vi "首页显示设置.vi"() -> ()   [LabVIEW 2016]
uses:
  <vilib>/Utility/config.llb/NI_LVConfig.lvlib
panel:
  in  "首页显示信息设置":T1={"水温"=FALSE, "pH"=FALSE, "DO"=FALSE, "Cond"=FALSE, "Turb"=FALSE, "氨氮"=FALSE, "总磷"=FALSE, "总氮"=FALSE, "CODMn"=FALSE, "CODCr"=FALSE, "水位"=FALSE, "流速"=FALSE, "瞬时流量"=FALSE, "室温"=TRUE, "湿度"=TRUE, "叶绿素a"=FALSE, "藻密度"=FALSE}
  in  "关闭":bool
  # "首页显示信息设置"
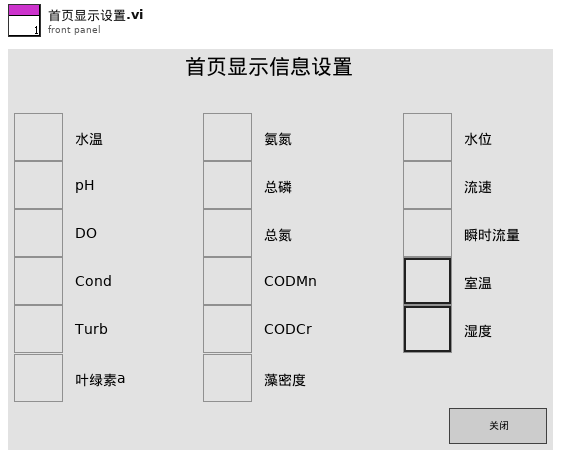
[diagram p1: front panel]
types:
  T1 = cluster{"水温":bool, "pH":bool, "DO":bool, "Cond":bool, "Turb":bool, "氨氮":bool, "总磷":bool, "总氮":bool, "CODMn":bool, "CODCr":bool, "水位":bool, "流速":bool, "瞬时流量":bool, "室温":bool, "湿度":bool, "叶绿素a":bool, "藻密度":bool}
  T2 = typedef "NI_LVConfig.lvlib/Config Data RefNum.ctl" = refnum<k1>
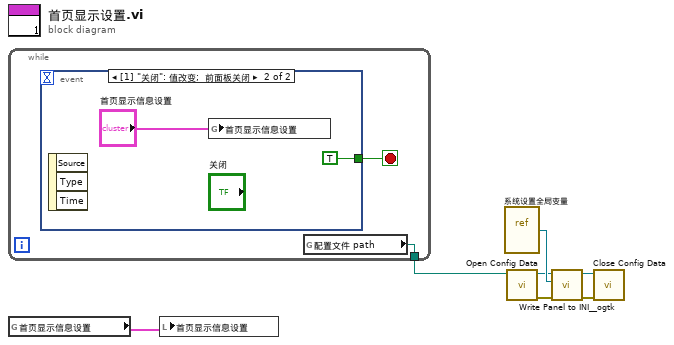
[diagram p0: block diagram]
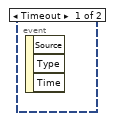
[diagram p2: hidden frame]
diagram:
  n1 = while {
    tunnel: [w8] -> w1
    stop <- w9 stop-if-true
    n2 = event shown="[1] \"关闭\": 值改变;  前面板关闭" {
      selector: _ -> [_ _]
      dyn-events: _ -> [_ _]
      timeout: _ -> [_ _]
      tunnel: [_ TRUE] -> w9
      event Timeout {
        n3 = event-data() -> ()  [unwired: 1 in, 3 out]
      }
      event "关闭": Value Change; Panel Close {
        n4 = event-data() -> ()  [unwired: 1 in, 3 out]
        n5 = global write "系统设置全局变量.vi" "首页显示信息设置"("首页显示信息设置") -> ()
      }
    }
    n6 = global read "ping全局.vi" "配置文件 path"() -> (w8:path)
  }
  n7 = global read "系统设置全局变量.vi" "首页显示信息设置"() -> (w2:T1)
  n8 = local write "首页显示信息设置"(w2) -> ()
  n9 = vi-ref "系统设置全局变量.vi"() -> (w4:refnum<vi>)
  n10 = call <vilib>:"Open Config Data.vi"("configuration file path"=w1) -> ("error out"=w6:errorcluster, "refnum"=w3:T2)  [unwired: 8 in, 1 out]
  n11 = call <userlib>:"Write Panel to INI__ogtk.vi"("error in (no error)"=w6, "VI ref"=w4, "refnum"=w3) -> ("error out"=w7:errorcluster, "refnum out"=w5:T2)  [unwired: 7 in]
  n12 = call <vilib>:"Close Config Data.vi"("error in (no error)"=w7, "refnum"=w5) -> ()  [unwired: 8 in, 2 out]
